vi "Load Into Sub Panel.vi"(8 "error in (no error)":errorcluster caption="错误输入（无错误）", 10 "VI引用":refnum<vi>, 11 "TPP demo V2 输入":refnum<class "TPP demo V2.lvclass">) -> (0 "error out":errorcluster caption="错误输出", 3 "TPP demo V2 输出":refnum<class "TPP demo V2.lvclass">)   [LabVIEW 2017, in "TPP demo V2.lvlib" / "TPP demo V2.lvclass"]
uses:
  TPP demo V2.lvclass
  TPP demo V2.lvclass/TPP demo V2.ctl
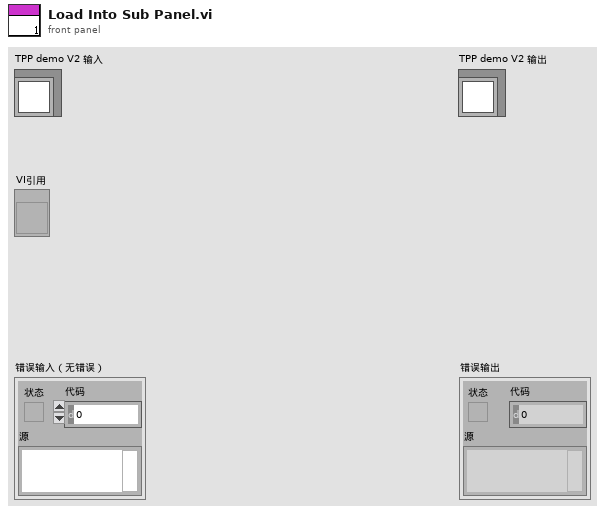
[diagram p1: front panel]
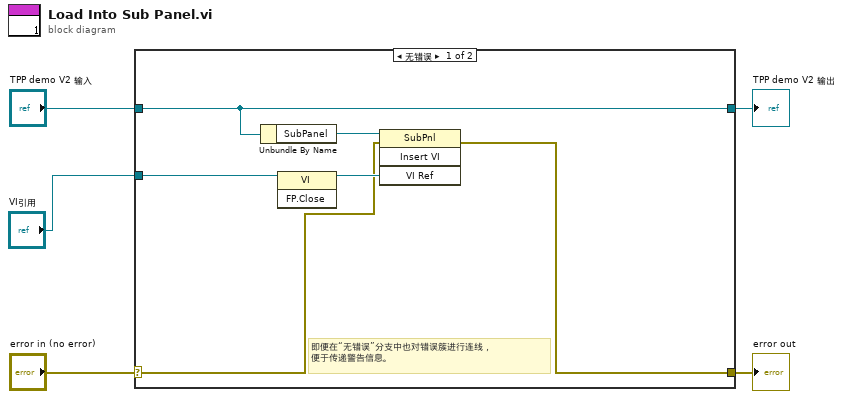
[diagram p0: block diagram]
diagram:
  n1 = case shown="无错误" "error in (no error)" {
    selector: "error in (no error)" -> [w7 w13]
    tunnel: [w6 w13] -> w4
    tunnel: [w11 w12] -> w2
    tunnel: "TPP demo V2 输入" -> [w11 w12]
    tunnel: "VI引用" -> [w9 _]
    frame No Error {
      # "即便在“无错误”分支中也对错误簇进行连线，\n便于传递警告信息。"
      n2 = Unbundle By Name(w11) -> ("SubPanel"=w10:refnum<vi>)
      n3 = invoke class="VI" method="FP.Close"(reference=w9) -> (reference out=w8:refnum<vi>)  [unwired: 2 in, 2 out]
      n4 = invoke class="SubPnl" method="Insert VI"(reference=w10, error in=w7, "VI Ref"=w8) -> (error out=w6:errorcluster)  [unwired: 1 in, 3 out]
    }
    frame Error {
    }
  }
  "error out" <- w4
  "TPP demo V2 输出" <- w2
